vi "CreatingandAccessingFile3.vi"() -> ()   [LabVIEW 2020]
panel:
  out "millisecond timer value":u32
  in  "milliseconds to wait":u32
  in  "stop":bool
  in  "file path (use dialog)":path
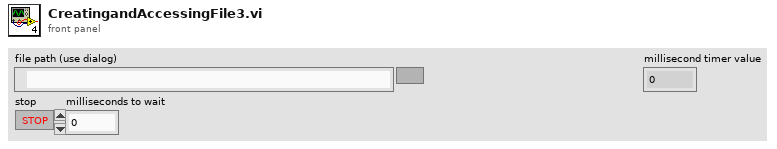
[diagram p1: front panel]
types:
  T1 = enum16{"open", "replace", "create", "open or create", "replace or create", "replace or create with confirmation"}
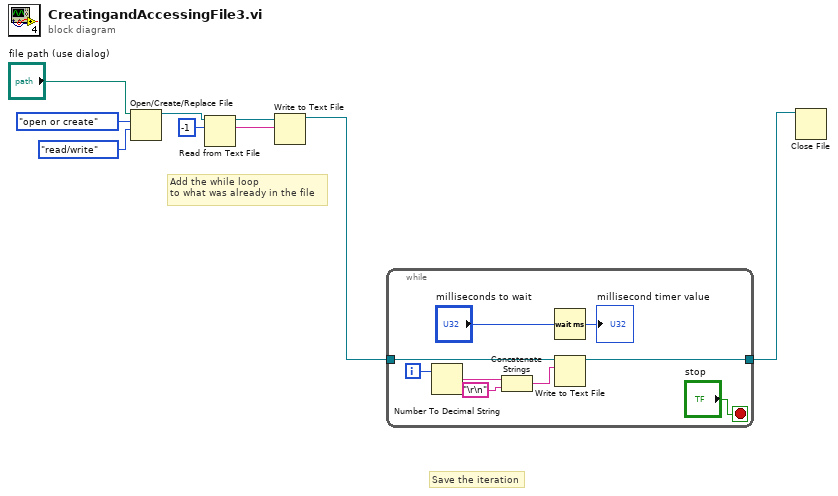
[diagram p0: block diagram]
diagram:
  # "Add the while loop \nto what was already in the file"
  # "Save the iteration"
  n1 = Open/Create/Replace File(file path (use dialog)="file path (use dialog)", operation (0:open)=T1."open or create", access (0:read/write)=enum16{"read/write", "read-only", "write-only"}."read/write") -> (refnum out=w5:refnum<file>)  [unwired: 3 in, 2 out]
  n2 = Read from Text File(file (use dialog)=w5, count=-1) -> (refnum out=w4:refnum<file>, text=w3:string)  [unwired: 2 in, 2 out]
  n3 = Write to Text File(file (use dialog)=w4, text=w3) -> (refnum out=w2:refnum<file>)  [unwired: 2 in, 2 out]
  n4 = while {
    tunnel: w2 -> [w18]
    tunnel: [w16] -> w6
    i -> [w17]
    stop <- "stop" stop-if-true
    n5 = Number To Decimal String(number=w17) -> (decimal integer string=w11:string)  [unwired: 1 in]
    n6 = Concatenate Strings(w11, "\r\n") -> (w10:string)
    n7 = Wait (ms)(milliseconds to wait="milliseconds to wait") -> (millisecond timer value=→"millisecond timer value":u32)
    n8 = Write to Text File(file (use dialog)=w18, text=w10) -> (refnum out=w16:refnum<file>)  [unwired: 2 in, 2 out]
  }
  n9 = Close File(refnum=w6) -> ()  [unwired: 1 in, 2 out]
